vi "get_ai_channel_name.vi"(10 "AI number":i8, 11 "DAQmx Device Name":tag) -> (3 "DAQmx Physical Channel":tag)   [LabVIEW 2024]
doc: "Creates a valid DAQmx Physical Channel name like Dev[x]/AI[y]\nDevice ID Dev[x] must be provided as DAQmx Device Name, analog input terminal name AI[y] is provided by an integer y at AI number."
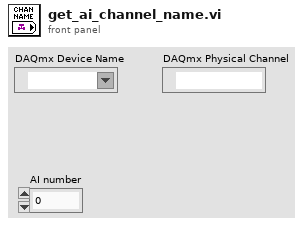
[diagram p1: front panel]
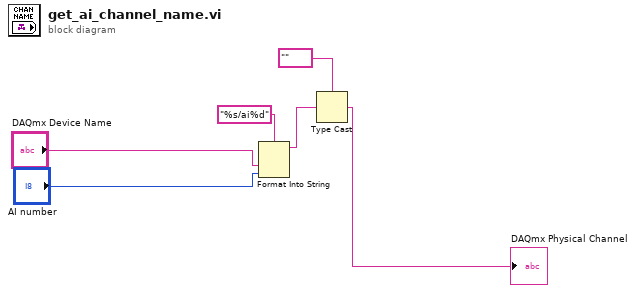
[diagram p0: block diagram]
diagram:
  n1 = Format Into String(format string="%s/ai%d", "DAQmx Device Name", "AI number") -> (resulting string=w5:string)  [unwired: 2 in, 1 out]
  n2 = Type Cast(type=tag "" ("DAQmx Physical Channel"), x=w5) -> (*(type *) &x=→"DAQmx Physical Channel":tag)
